vi "Network control test 2 writer.vi"() -> ()   [LabVIEW 2018]
uses:
  <vilib>/dex/Stream Element Allocation Mode.ctl
panel:
  in  "Stop Button":bool
  out "number (0 to 1)":dbl
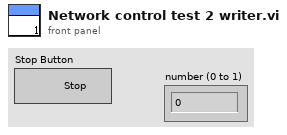
[diagram p1: front panel]
types:
  T1 = typedef "Stream Element Allocation Mode.ctl" = u32
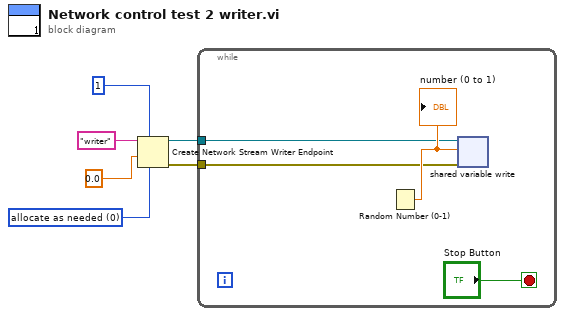
[diagram p0: block diagram]
diagram:
  w5 = T1 0 items=["allocate as needed", "pre-allocate"] ("element allocation mode")
  n1 = Create Network Stream Writer Endpoint(6:w5, 7:1 ("writer buffer size"), 9:0.0, 11:"writer" ("writer name")) -> (0:w1:errorcluster, 3:w2:refnum<k21>)  [unwired: 3 in]
  n2 = while {
    tunnel: w2 -> [w8]
    tunnel: w1 -> [w7]
    stop <- "Stop Button" stop-if-true
    n3 = Random Number (0-1)() -> (number: 0 to 1=w10:dbl)
    "number (0 to 1)" <- w10
    n4 = shared-variable-write(w8, w7, w10) -> ()  [unwired: 1 in, 3 out]
  }
